vi "corr.vi"(9 "Enum":T1(ring), 10 "Orden":T2(array[ring])=[enum."espejos", enum."voltaje", enum."polarizador", enum."potenciometro "], 11 "Numeric":i32) -> (2 "Enum 2":T1(ring))   [LabVIEW 2016]
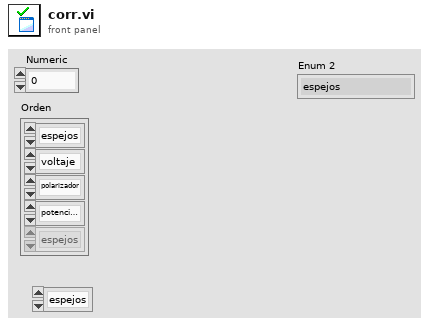
[diagram p1: front panel]
types:
  T1 = enum16{"espejos", "polarizador", "voltaje", "potenciometro ", "CCD", "lockin", "laser", "ninguno"}
  T2 = enum16{"espejos", "polarizador", "voltaje", "potenciometro ", "CCD", "lockin", "laser", "ninguno"}[]
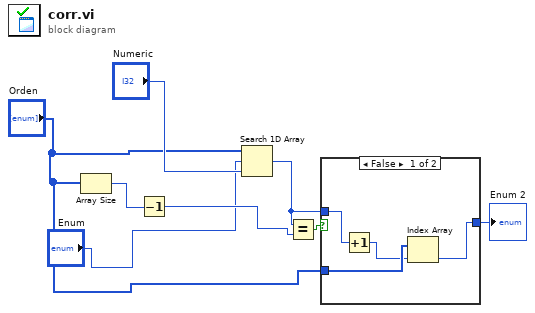
[diagram p0: block diagram]
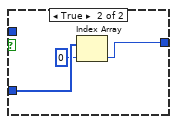
[diagram p2: hidden frame]
diagram:
  n1 = Array Size(array="Orden") -> (size(s)=w8:i32)
  n2 = Decrement(x=w8) -> (x-1=w6:i32)
  n3 = Search 1D Array(1D array="Orden", element="Enum", start index (0)="Numeric") -> (index of element=w5:i32)
  n4 = Equal?(x=w5, y=w6) -> (x = y?=w7:bool)
  n5 = case shown="False" w7 {
    tunnel: [w9 w13] -> w1
    tunnel: "Orden" -> [w12 w15]
    tunnel: w5 -> [w11 _]
    frame False {
      n6 = Increment(x=w11) -> (x+1=w10:i32)
      n7 = Index Array(array=w12, index=w10) -> (element=w9:T1)
    }
    frame True {
      n8 = Index Array(array=w15, index=0) -> (element=w13:T1)
    }
  }
  "Enum 2" <- w1
